vi "FPWindowStateSetting(SubVI).vi"(8 "Error In":errorcluster, 11 "Enum in":refnum<vi>) -> (0 "Error Out":errorcluster)   [LabVIEW 2018]
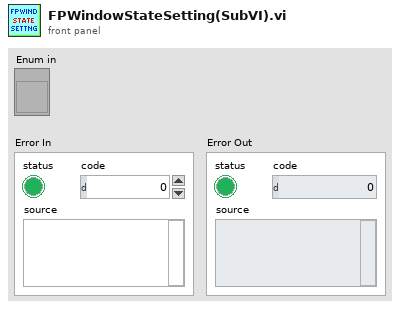
[diagram p1: front panel]
types:
  T1 = enum16{"Standart", "Closed", "Hidden", "Minimized", "Maximized", "Invalid"}
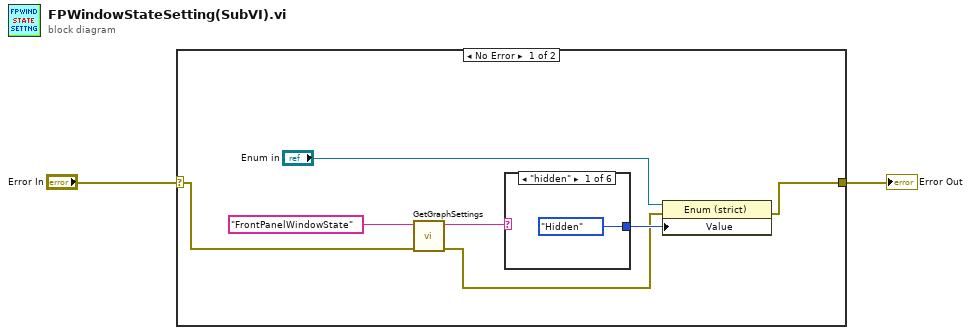
[diagram p0: block diagram]
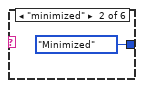
[diagram p2: hidden frame]
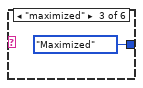
[diagram p3: hidden frame]
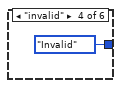
[diagram p4: hidden frame]
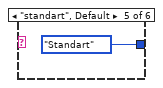
[diagram p5: hidden frame]
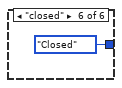
[diagram p6: hidden frame]
diagram:
  n1 = case shown="No Error" "Error In" {
    selector: "Error In" -> [w5 w16]
    tunnel: [w3 w16] -> w1
    frame No Error {
      n2 = call "GetGraphSettings.vi"("Error In"=w5, "Setting's name"="FrontPanelWindowState") -> ("Error Out"=w4:errorcluster, "Result"=w7:string)  [unwired: 8 in]
      n3 = case shown="\"hidden\"" w7 {
        tunnel: [T1."Hidden" ("Value") T1."Minimized" ("Value") T1."Maximized" ("Value") T1."Invalid" ("Value") T1."Standart" ("Value") T1."Closed" ("Value")] -> w6
        frame "hidden" {
        }
        frame "minimized" {
        }
        frame "maximized" {
        }
        frame "invalid" {
        }
        frame "standart", Default {
        }
        frame "closed" {
        }
      }
      n4 = property on="Property Node" class="Enum (strict)"(reference="Enum in", error in=w4, "Value"=w6) -> (error out=w3:errorcluster)  [unwired: 1 out]
    }
    frame Error {
    }
  }
  "Error Out" <- w1
